vi "get_wl_(serial).vi"(8 "error in (no error)":errorcluster, 10 "max_attempts":i32=10) -> (0 "error out":errorcluster, 2 "ch2":dbl format="%#_9g", 3 "ch1":dbl format="%#_9g")   [LabVIEW 2017, in "highfinesse.lvlib"]
uses:
  <vilib>/Instr/_visa.llb/VISA Configure Serial Port (Instr).vi
  highfinesse.lvlib
panel:
  out "attempts":i32
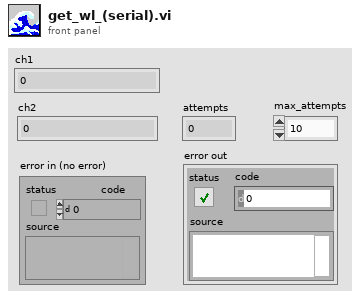
[diagram p1: front panel]
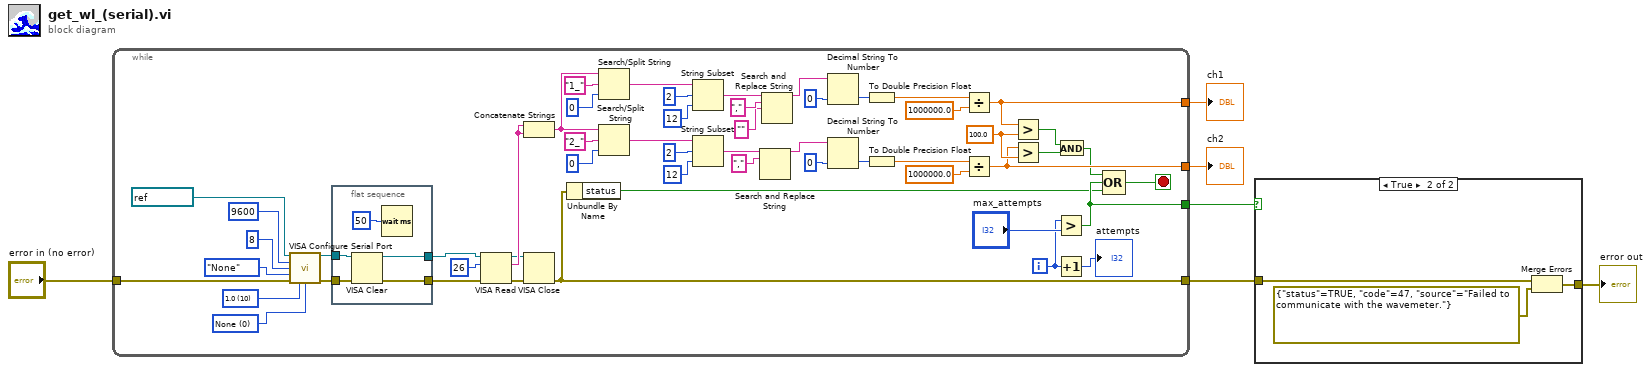
[diagram p0: block diagram]
diagram:
  n1 = while {
    tunnel: [w20] -> w6
    tunnel: [w21] -> w5
    tunnel: "error in (no error)" -> [w19]
    tunnel: [w14] -> w2
    tunnel: [w15] -> w3
    i -> [w8]
    stop <- w16 stop-if-true
    w26 = 100.0 ("y")
    w55 = u16 0 items=["None", "XON/XOFF", "RTS/CTS", "XON/XOFF & RTS/CTS", "DTR/DSR", "XON/XOFF & DTR/DSR"] ("flow control (0:none)")
    w56 = u16 10 items=["1.0"=10, "1.5"=15, "2.0"=20] ("stop bits (10: 1 bit)")
    n2 = call-poly "VISA Configure Serial Port"("VISA resource name"=refnum<visa-resource-name> "COM6", "baud rate (9600)"=u32 9600, "data bits (8)"=u16 8, "parity (0:none)"=enum16{"None", "Odd", "Even", "Mark", "Space"}."None", "error in (no error)"=w19, "stop bits (10: 1 bit)"=w56, "flow control (0:none)"=w55) -> ("VISA resource name out"=w12:refnum<visa-resource-name>, "error out"=w9:errorcluster)  [unwired: 7 in]
    n3 = flat-sequence {
      tunnel: w12 -> [w64]
      tunnel: [w63] -> w11
      tunnel: [w62] -> w10
      tunnel: w9 -> [w61]
      frame #0 {
        n4 = VISA Clear(VISA resource name=w64, error in (no error)=w61) -> (VISA resource name out=w63:refnum<visa-resource-name>, error out=w62:errorcluster)
        n5 = Wait (ms)(milliseconds to wait=u32 50) -> ()  [unwired: 1 out]
      }
    }
    n6 = VISA Read(VISA resource name=w11, byte count=u32 26, error in (no error)=w10) -> (VISA resource name out=w23:refnum<visa-resource-name>, read buffer=w53:string, error out=w22:errorcluster)  [unwired: 1 out]
    n7 = Concatenate Strings(w53, w53) -> (w44:string)
    n8 = VISA Close(VISA resource name=w23, error in (no error)=w22) -> (error out=w14:errorcluster)
    n9 = Unbundle By Name(w14) -> ("status"=w13:bool)
    n10 = Search/Split String(string=w44, search string/char (-)="1_", offset (0)=0) -> (match + rest of string=w50:string)  [unwired: 2 out]
    n11 = Search/Split String(string=w44, search string/char (-)="2_", offset (0)=0) -> (match + rest of string=w46:string)  [unwired: 2 out]
    n12 = String Subset(string=w50, offset (0)=2, length (rest)=12 ("length (rest)")) -> (substring=w34:string)
    n13 = String Subset(string=w46, offset (0)=2, length (rest)=12 ("length (rest)")) -> (substring=w27:string)
    n14 = Search and Replace String(input string=w27, search string=",") -> (result string=w32:string)  [unwired: 6 in, 3 out]
    n15 = Search and Replace String(input string=w34, search string=",", replace string="" ("replace string (\"\")")) -> (result string=w39:string)  [unwired: 5 in, 3 out]
    n16 = Decimal String To Number(string=w39, default (0L)=0 ("default (0 I32)")) -> (number=w37:i32)  [unwired: 1 in, 1 out]
    n17 = Decimal String To Number(string=w32, default (0L)=0 ("default (0 I32)")) -> (number=w30:i32)  [unwired: 1 in, 1 out]
    n18 = To Double Precision Float(number=w37) -> (double precision float=w36:dbl)
    n19 = To Double Precision Float(number=w30) -> (double precision float=w29:dbl)
    n20 = Divide(x=w36, y=1000000.0) -> (x/y=w20:dbl)
    n21 = Divide(x=w29, y=1000000.0) -> (x/y=w21:dbl)
    n22 = Greater?(x=w20, y=w26) -> (0:w25:bool)
    n23 = Greater?(x=w21, y=w26) -> (0:w24:bool)
    n24 = Greater?(x=w8, y="max_attempts") -> (0:w15:bool)
    n25 = Increment(x=w8) -> (x+1=→"attempts":i32)
    n26 = And(x=w25, y=w24) -> (x .and. y?=w17:bool)
    n27 = Compound Arithmetic op=OR(w17, w15, w13) -> (w16:bool)
  }
  "ch1" <- w6
  "ch2" <- w5
  n28 = case shown="True" w3 {
    tunnel: w2 -> [w66 w69]
    tunnel: [w66 w68] -> w1
    frame False {
    }
    frame True {
      n29 = Merge Errors(w69, errorcluster {"status"=TRUE, "code"=47, "source"="Failed to communicate with the wavemeter."} ("error in")) -> (w68:errorcluster)
    }
  }
  "error out" <- w1
